vi "W vs Z main4g.vi"() -> ()   [LabVIEW 2016]
panel:
  out "cursor X's":dbl[](array[numeric])
  out "Contains waist?":bool[](array[boolean])
  out "FWHM":dbl[](array[numeric])
  out "min w":dbl[](array[numeric])
  out "min z":dbl[](array[numeric])
  out "w Matrix":dbl[][](array[numeric])
  out "Z Matrix":dbl[][](array[numeric])
  out "Number of lenses":i32
  in  "Lens Focal lengths":dbl[](array[numeric]) format="%.3f"
  in  "FWHM(T)?":bool
  out "Cursor List":T1(array[cluster]) {"Location"."Y" format="%.2f"; "Location"."X" format="%.2f"}
  in  "z stop":dbl=1000.0 format="%.2f"
  in  "N steps":i32=500
  out "Q start":cdb format="%.4f"
  out "W vs Z":cluster{dbl[], dbl[]}[](graph)
  in  "beam radius(w)":dbl=0.6 format="%.5f"
  in  "Radius of Curvature":dbl=inf format="%.2f"
  in  "Wavelength":dbl=0.00035 format="%.6f"
  in  "z start":dbl format="%.2f"
  # "All values are entered in mm"
  # "w is the 1/e field radius"
  # "w x 1.18 to get FWHM of the Intensity"
  # "Zs plotted above. Each row is a segment between adjacent lenses"
  # "Ws plotted above. Each row is a segment between adjacent lenses"
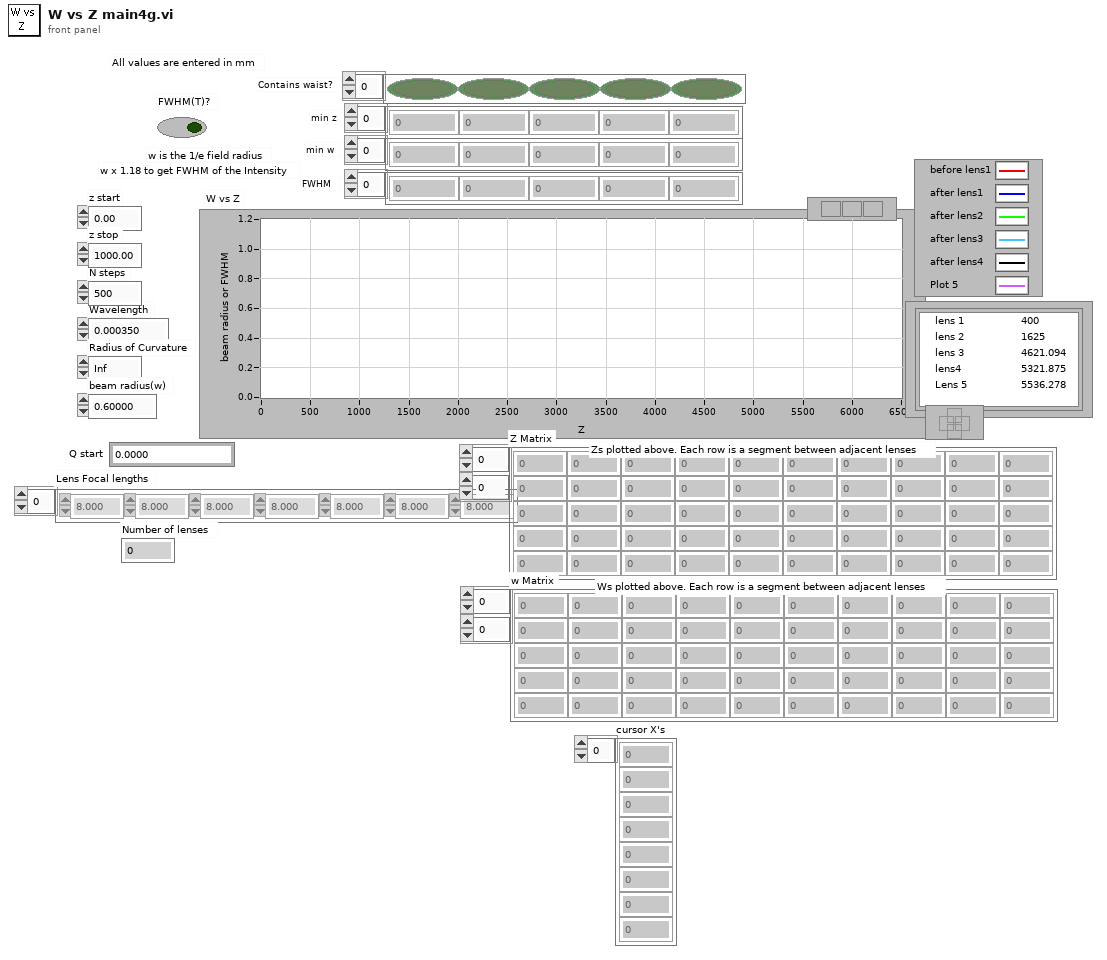
[diagram p1: front panel]
types:
  T1 = cluster{"Name":string, "Color":u32, "Hair Style":u8, "Point Style":u8, "Name Visible":bool, "Trackable":bool, "Lock Style":u32, "Plot Number":u32, "Marker Index":i32, "Location":cluster{"X":dbl, "Y":dbl}}[]
  T2 = cluster{"Name":string, "Color":u32, "Style":u8, "Point Style":u8, "Name Visible":bool, "Allow Drag":bool, "Lock Style":u32, "Plot":u32, "Index":i32, "Position":cluster{"X":dbl, "Y":dbl}}[]
  T3 = cluster{"Name":string, "Color":u32, "Style":u8, "Point Style":u8, "Name Visible":bool, "Allow Drag":bool, "Lock Style":u32, "Plot":u32, "Index":i32, "Position":cluster{"X":dbl, "Y":dbl}}
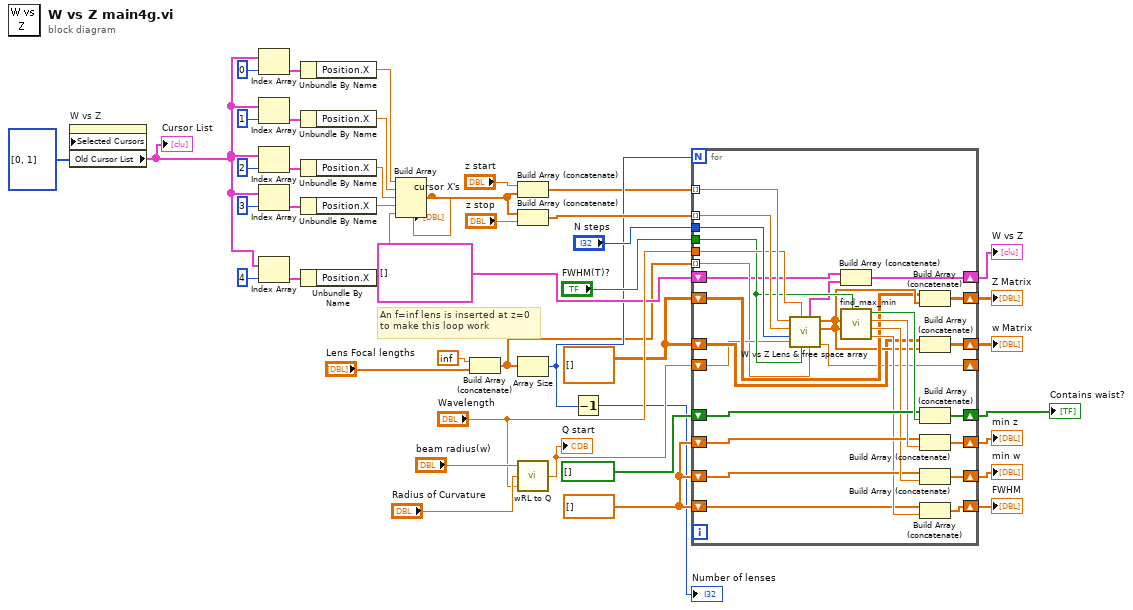
[diagram p0: block diagram]
diagram:
  w12 = dbl[] []
  w11 = dbl[][] []
  # "An f=inf lens is inserted at z=0\nto make this loop work"
  n1 = property on="W vs Z" class="XYGraph (strict)"("Selected Cursors"=u32[] [0, 1]) -> ("Old Cursor List"=w3:T2)  [unwired: 2 in, 2 out]
  "Cursor List" <- w3
  n2 = Index Array(array=w3, index=0 ("Index")) -> (element=w41:T3)
  n3 = Index Array(array=w3, index=1 ("Index")) -> (element=w39:T3)
  n4 = Index Array(array=w3, index=2 ("Index")) -> (element=w35:T3)
  n5 = Index Array(array=w3, index=3 ("Index")) -> (element=w33:T3)
  n6 = Index Array(array=w3, index=4 ("Index")) -> (element=w4:T3)
  n7 = Unbundle By Name(w41) -> ("Position.X"=w14:dbl)
  n8 = Unbundle By Name(w39) -> ("Position.X"=w28:dbl)
  n9 = Unbundle By Name(w35) -> ("Position.X"=w26:dbl)
  n10 = Unbundle By Name(w33) -> ("Position.X"=w25:dbl)
  n11 = Unbundle By Name(w4) -> ("Position.X"=w2:dbl)
  n12 = Build Array(w14, w28, w26, w25, w2) -> (w5:dbl[])
  "cursor X's" <- w5
  n13 = Build Array (concatenate)(inf, "Lens Focal lengths") -> (w15:dbl[])
  n14 = Build Array (concatenate)("z start", w5) -> (w6:dbl[])
  n15 = Build Array (concatenate)(w5, "z stop") -> (w27:dbl[])
  n16 = Array Size(array=w15) -> (size(s)=w18:i32)
  n17 = call "wRL to Q.vi"("Wavelength"="Wavelength", "Radius of Curvature"="Radius of Curvature", "beam radius(w)"="beam radius(w)") -> ("Q"=w13:cdb)
  "Q start" <- w13
  n18 = Decrement(x=w18) -> (x-1=→"Number of lenses":i32)
  n19 = for {
    N: w18 -> [_]
    tunnel: "N steps" -> [w73]
    tunnel: w27 -> [w72] mode=indexing
    tunnel: w6 -> [w71] mode=indexing
    tunnel: "Wavelength" -> [w70]
    tunnel: "FWHM(T)?" -> [w69]
    shift-right: [w68] -> w8
    shift-left: bool[] [] -> [w66]
    shift-right: [w64] -> w22
    shift-left: w12 -> [w63]
    shift-right: [w61] -> w21
    shift-left: w12 -> [w60]
    shift-right: [w48] -> w20
    shift-left: w12 -> [w58]
    shift-right: [w56] -> w29
    shift-left: w11 -> [w55]
    shift-right: [w53] -> w23
    shift-left: w11 -> [w52]
    shift-right: [w51] -> _
    shift-left: w13 -> [w50]
    tunnel: w15 -> [w49] mode=indexing
    shift-right: [w46] -> w30
    shift-left: cluster{dbl[], dbl[]}[] [] -> [w45]
    n20 = call "W vs Z Lens & free space array.vi"("lens focal length"=w49, "FWHM(T)?"=w69, "Wavelength"=w70, "Q in"=w50, "N steps"=w73, "z stop"=w72, "z start"=w71) -> ("Q out"=w51:cdb, "w/FWHM Array"=w54:dbl[], "Z Array"=w57:dbl[], "W/FWHM vs Z"=w47:cluster{dbl[], dbl[]})  [unwired: 1 out]
    n21 = Build Array (concatenate)(w45, w47) -> (w46:cluster{dbl[], dbl[]}[])
    n22 = call "find_max_min.vi"("FWHM(T)?"=w69, "w Array"=w54, "z Array"=w57) -> ("FWHM"=w59:dbl, "min w"=w62:dbl, "min  z"=w65:dbl, "contains waist?"=w67:bool)  [unwired: 5 in]
    n23 = Build Array (concatenate)(w55, w57) -> (w56:dbl[][])
    n24 = Build Array (concatenate)(w52, w54) -> (w53:dbl[][])
    n25 = Build Array (concatenate)(w66, w67) -> (w68:bool[])
    n26 = Build Array (concatenate)(w63, w65) -> (w64:dbl[])
    n27 = Build Array (concatenate)(w60, w62) -> (w61:dbl[])
    n28 = Build Array (concatenate)(w58, w59) -> (w48:dbl[])
  }
  "W vs Z" <- w30
  "Z Matrix" <- w29
  "w Matrix" <- w23
  "min z" <- w22
  "min w" <- w21
  "FWHM" <- w20
  "Contains waist?" <- w8
